vi "GoToNearestMultiple.vi"(2 "Multiple":dbl=360.0, 7 "Numeric":dbl) -> (8 "Snapped Numeric":dbl)   [LabVIEW 2016]
doc: "This VI takes the input and rounds it to the nearest multiple.\n\nCreated by Team 4130 for use in the 2016-2017 FRC season"
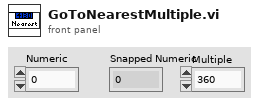
[diagram p1: front panel]
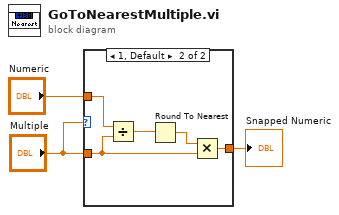
[diagram p0: block diagram]
diagram:
  n1 = case shown="1, Default" "Multiple" {
    tunnel: [w4 w9] -> w3
    tunnel: "Numeric" -> [w4 w6]
    tunnel: "Multiple" -> [_ w5]
    frame 0 {
    }
    frame 1, Default {
      n2 = Divide(x=w6, y=w5) -> (x/y=w7:dbl)
      n3 = Round To Nearest(number=w7) -> (nearest integer value=w8:dbl)
      n4 = Multiply(x=w8, y=w5) -> (x*y=w9:dbl)
    }
  }
  "Snapped Numeric" <- w3
